vi "Prober_MoveToHome.vi"(8 "error in (no error)":errorcluster, 11 "SemiProbe in":refnum<class "SemiProbe.lvclass">) -> (0 "error out":errorcluster, 3 "SemiProbe out":refnum<class "SemiProbe.lvclass">)   [LabVIEW 2013, in "SemiProbe.lvclass"]
uses:
  SemiProbe.lvclass
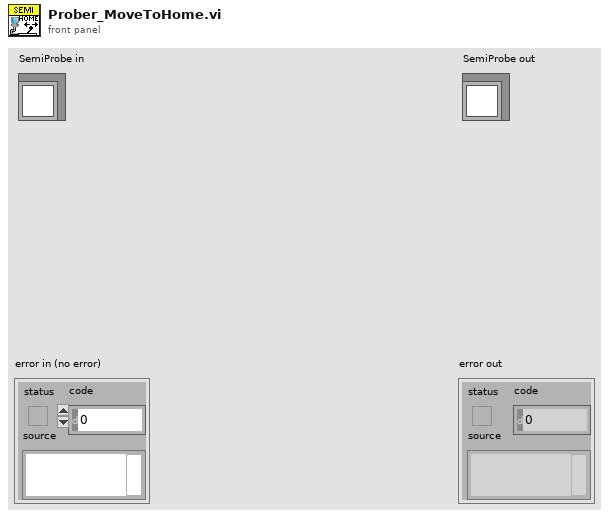
[diagram p1: front panel]
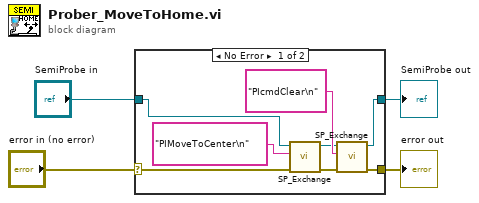
[diagram p0: block diagram]
diagram:
  n1 = case shown="No Error" "error in (no error)" {
    selector: "error in (no error)" -> [w5 w13]
    tunnel: "SemiProbe in" -> [w8 w14]
    tunnel: [w7 w14] -> w2
    tunnel: [w6 w13] -> w1
    frame No Error {
      n2 = call-dynamic "SP_Exchange.vi"("error in (no error)"=w5, "command"="PIMoveToCenter\n" ("Error String IN"), "SemiProbe in"=w8) -> ("error out"=w10:errorcluster, "SemiProbe out"=w9:refnum<class "SemiProbe.lvclass">)  [unwired: 4 in, 3 out]
      n3 = call-dynamic "SP_Exchange.vi"("error in (no error)"=w10, "command"="PIcmdClear\n" ("Error String IN"), "SemiProbe in"=w9) -> ("error out"=w6:errorcluster, "SemiProbe out"=w7:refnum<class "SemiProbe.lvclass">)  [unwired: 4 in, 3 out]
    }
    frame Error {
    }
  }
  "error out" <- w1
  "SemiProbe out" <- w2
